vi "CalibrateSingleAxis.vi"(5 "Numeric":i32, 6 "beam detection para":T1 {"smal para"."Measurement Parameter" items=["Center of Mass X", "Center of Mass Y", "First Pixel X", "First Pixel Y", "Bounding Rect Left", "Bounding Rect Top", "Bounding Rect Right", "Bounding Rect Bottom", "Max Feret Diameter Start X", "Max Feret Diameter Start Y", "Max Feret Diameter End X", "Max Feret Diameter End Y", "Max Horiz. Segment Length Left", "Max Horiz. Segment Length Right", "Max Horiz. Segment Length Row", "-", "Bounding Rect Width", "Bounding Rect Height", "Bounding Rect Diagonal", "Perimeter", "Convex Hull Perimeter", "Holes' Perimeter", "Max Feret Diameter", "Equivalent Ellipse Major Axis", "Equivalent Ellipse Minor Axis", "Equivalent Ellipse Minor Axis (Feret)", "Equivalent Rect Long Side", "Equivalent Rect Short Side", "Equivalent Rect Diagonal", "Equivalent Rect Short Side (Feret)", "Average Horiz. Segment Length", "Average Vert. Segment Length", "Hydraulic Radius", "Waddel Disk Diameter", "-", "Area", "Holes' Area", "Particle & Holes' Area", "Convex Hull Area", "Image Area", "-", "Number of Holes", "Number of Horiz. Segments", "Number of Vert. Segments", "-", "Orientation", "Max Feret Diameter Orientation", "-", "% Area/Image Area", "% Area/(Particle & Holes' Area)", "Ratio of Equivalent Ellipse Axes", "Ratio of Equivalent Rect Sides", "-", "Elongation Factor", "Compactness Factor", "Heywood Circularity Factor", "Type Factor", "-", "Sum X", "Sum Y", "Sum XX", "Sum XY", "Sum YY", "Sum XXX", "Sum XXY", "Sum XYY", "Sum YYY", "-", "Moment of Inertia XX", "Moment of Inertia XY", "Moment of Inertia YY", "Moment of Inertia XXX", "Moment of Inertia XXY", "Moment of Inertia XYY", "Moment of Inertia YYY", "Norm. Moment of Inertia XX", "Norm. Moment of Inertia XY", "Norm. Moment of Inertia YY", "Norm. Moment of Inertia XXX", "Norm. Moment of Inertia XXY", "Norm. Moment of Inertia XYY", "Norm. Moment of Inertia YYY", "Hu Moment 1", "Hu Moment 2", "Hu Moment 3", "Hu Moment 4", "Hu Moment 5", "Hu Moment 6", "Hu Moment 7"]; "smal para"."Range Lower Value" format="%.2f"; "smal para"."Range Upper Value" format="%.2f"; "detection method" items=["clustering", "entropy", "metric", "moments", "inter-class variance"]; "Filter" items=["No Filter", "Median Filter", "Low Pass Filter"]}, 8 "error in (no error)":errorcluster, 9 "RelativeSettings.Axis 1":refnum<vi>[](array[refnum]), 10 "RelativeMove.Axis 1":refnum<vi>[](array[refnum]), 11 "Refnum in":T3) -> (0 "Axis Inverted":bool, 1 "slope":dbl, 3 "accepted":bool, 4 "error out":errorcluster)   [LabVIEW 2013]
uses:
  <vilib>/vision/Image Controls.llb/IMAQ Image.ctl
  Ctrs/beam detection.ctl
  <vilib>/Analysis/NI_AALPro.lvlib
panel:
  out "slope 2":dbl
  out "slope 1":dbl
  out "live":cluster{dbl[], "Best Linear Fit":dbl[]}[](graph)
  out "XY Graph":cluster{dbl[], "Best Linear Fit":dbl[]}[](graph)
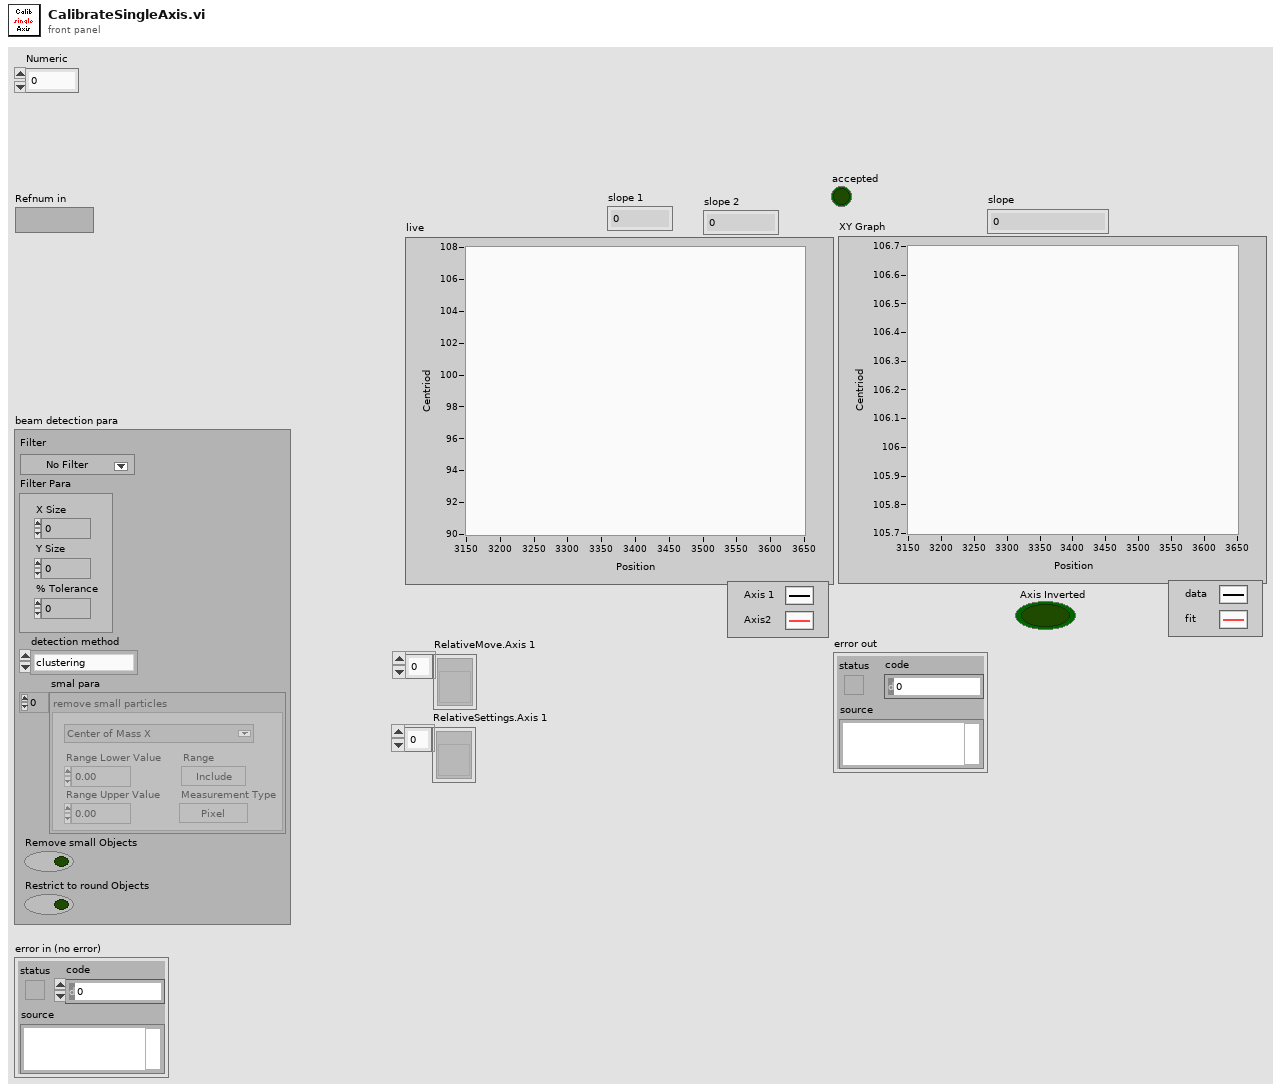
[diagram p1: front panel]
types:
  T1 = typedef "beam detection.ctl" = cluster{"Filter":u16, "Filter Para":cluster{"X Size":i32, "Y Size":i32, "% Tolerance":i32}, "detection method":i32, "smal para":cluster{"Measurement Parameter":T2, "Range Lower Value":dbl, "Range Upper Value":dbl, "Range":bool, "Measurement Type":bool}[], "Remove small Objects":bool, "Restrict to round Objects":bool}
  T2 = typedef "Particle Parameters" = i32
  T3 = typedef "IMAQ Image.ctl" = refnum<image>
  T4 = cluster{"Position":dbl[], "Best Linear Fit":dbl[]}
  T5 = cluster{"Position":dbl[], "Best Linear Fit":dbl[]}[]
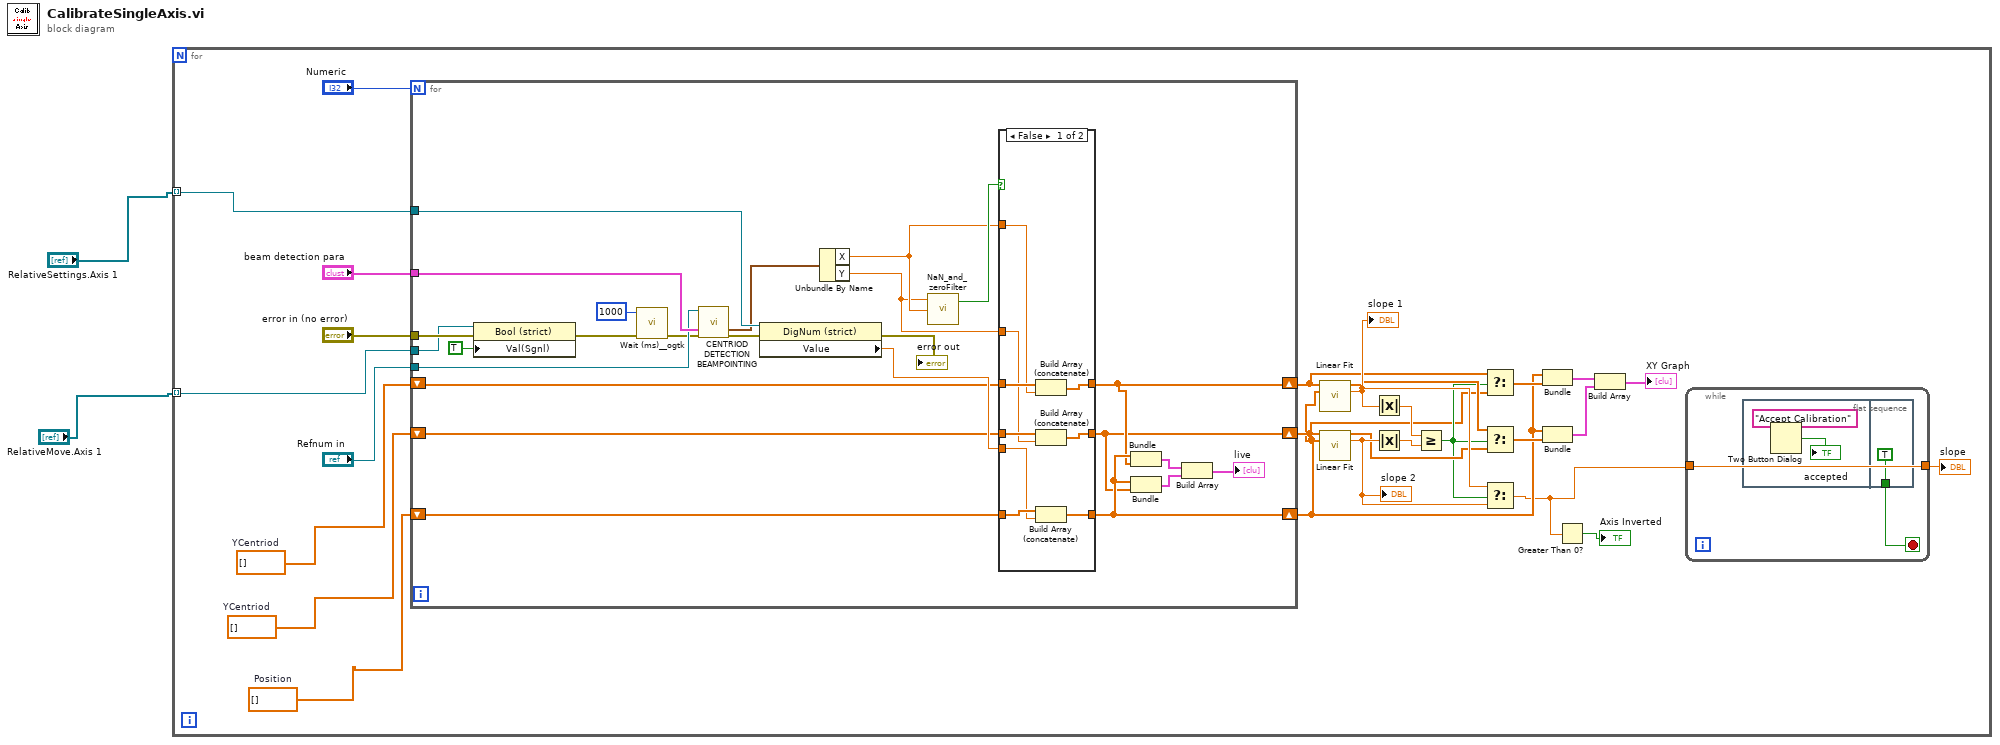
[diagram p0: block diagram]
diagram:
  n1 = for {
    tunnel: "RelativeMove.Axis 1" -> [w8] mode=indexing
    tunnel: "RelativeSettings.Axis 1" -> [w7] mode=indexing
    w3 = dbl[] []  # Position
    w4 = dbl[] []  # YCentriod
    w5 = dbl[] []  # YCentriod
    n2 = for {
      N: "Numeric" -> [_]
      tunnel: "beam detection para" -> [w58]
      tunnel: "error in (no error)" -> [w57]
      tunnel: w8 -> [w56]
      tunnel: "Refnum in" -> [w55]
      tunnel: w7 -> [w52]
      shift-right: [w40] -> w6
      shift-left: w5 -> [w44]
      shift-right: [w39] -> w13
      shift-left: w4 -> [w43]
      shift-right: [w41] -> w12
      shift-left: w3 -> [w42]
      n3 = property class="Bool (strict)"(reference=w56, error in=w57, "Val(Sgnl)"=TRUE ("Value (Signaling)")) -> (error out=w54:errorcluster)  [unwired: 1 out]
      n4 = call <userlib>:"Wait (ms)__ogtk.vi"("error in (no error)"=w54, "milliseconds to wait"=1000 ("Value")) -> ("error out"=w53:errorcluster)  [unwired: 8 in, 1 out]
      n5 = call "CENTRIOD DETECTION BEAMPOINTING.vi"("Refnum in"=w55, "beam detection para"=w58, "error in (no error)"=w53) -> ("Centriod"=w50:cluster{"X":dbl, "Y":dbl}, "error out"=w51:errorcluster)  [unwired: 10 in, 5 out]
      n6 = property class="DigNum (strict)"(reference=w52, error in=w51) -> (error out=→"error out":errorcluster, "Value"=w45:dbl)  [unwired: 1 out]
      n7 = Unbundle By Name(w50) -> ("X"=w47:dbl, "Y"=w46:dbl)
      n8 = call "NaN_and_zeroFilter.vi"("X"=w47, "Y"=w46) -> ("NaNor0"=w48:bool)  [unwired: 2 in]
      n9 = case shown="False" w48 {
        tunnel: w47 -> [w67 _]
        tunnel: w46 -> [w64 _]
        tunnel: w45 -> [w61 _]
        tunnel: w44 -> [w68 w71]
        tunnel: [w66 w71] -> w40
        tunnel: w43 -> [w65 w70]
        tunnel: [w63 w70] -> w39
        tunnel: w42 -> [w62 w69]
        tunnel: [w60 w69] -> w41
        frame False {
          n10 = Build Array (concatenate)(w68, w67) -> (w66:dbl[])
          n11 = Build Array (concatenate)(w65, w64) -> (w63:dbl[])
          n12 = Build Array (concatenate)(w62, w61) -> (w60:dbl[])
        }
        frame True {
        }
      }
      n13 = Bundle("Position"=w41, "YCentriod"=w40) -> (w37:cluster{"Position":dbl[], "YCentriod":dbl[]})  [unwired: 1 in]
      n14 = Bundle("Position"=w41, "YCentriod"=w39) -> (w36:cluster{"Position":dbl[], "YCentriod":dbl[]})  [unwired: 1 in]
      n15 = Build Array(w37, w36) -> (→"live":cluster{"Position":dbl[], "YCentriod":dbl[]}[])
    }
    n16 = call <vilib>:"Linear Fit.vi"("Y"=w6, "X"=w12) -> ("Best Linear Fit"=w21:dbl[], "slope"=w23:dbl)  [unwired: 9 in, 3 out]
    "slope 1" <- w23
    n17 = call <vilib>:"Linear Fit.vi"("Y"=w13, "X"=w12) -> ("Best Linear Fit"=w20:dbl[], "slope"=w22:dbl)  [unwired: 9 in, 3 out]
    "slope 2" <- w22
    n18 = Absolute Value(x=w23) -> (abs(x)=w25:dbl)
    n19 = Absolute Value(x=w22) -> (abs(x)=w24:dbl)
    n20 = Greater Or Equal?(x=w25, y=w24) -> (x >= y?=w19:bool)
    n21 = Select(t=w6, s=w19, f=w13) -> (s? t:f=w18:dbl[])
    n22 = Select(t=w21, s=w19, f=w20) -> (s? t:f=w17:dbl[])
    n23 = Select(t=w23, s=w19, f=w22) -> (s? t:f=w10:dbl)
    n24 = Bundle("Position"=w12, "YCentriod"=w18) -> (w16:cluster{"Position":dbl[], "YCentriod":dbl[]})  [unwired: 1 in]
    n25 = Bundle("Position"=w12, "Best Linear Fit"=w17) -> (w15:T4)  [unwired: 1 in]
    n26 = Greater Than 0?(x=w10) -> (x > 0?=→"Axis Inverted":bool)
    n27 = Build Array(w16, w15) -> (→"XY Graph":T5)
    n28 = while {
      tunnel: w10 -> [w31]
      tunnel: [w31] -> w9
      stop <- w30 stop-if-true
      n29 = flat-sequence {
        tunnel: [TRUE] -> w30
        frame #0 {
          n30 = Two Button Dialog(message="Accept Calibration") -> (T button?=→"accepted":bool)  [unwired: 2 in]
        }
        frame #1 {
        }
      }
    }
    "slope" <- w9
  }
